vi "UDP dSpace Reveiver.vi"(7 "milliseconds to wait":u32, 8 "error in (no error)":errorcluster, 10 "ENQUE DIRECTLY":refnum<queue>, 11 "UDP Network Connection in":refnum<k16>) -> (0 "error out":errorcluster)   [LabVIEW 2016]
uses:
  Globale Variablen VI/AutonomousMode.vi
  Globale Variablen VI/Global Variables.vi
panel:
  out "value":u32
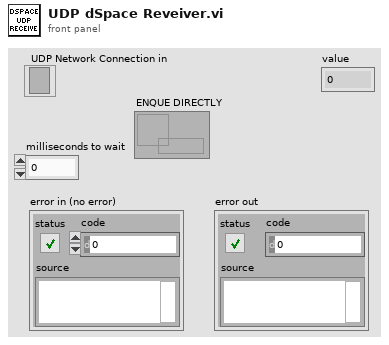
[diagram p1: front panel]
types:
  T1 = enum16{"big-endian, network order", "native, host order", "little-endian"}
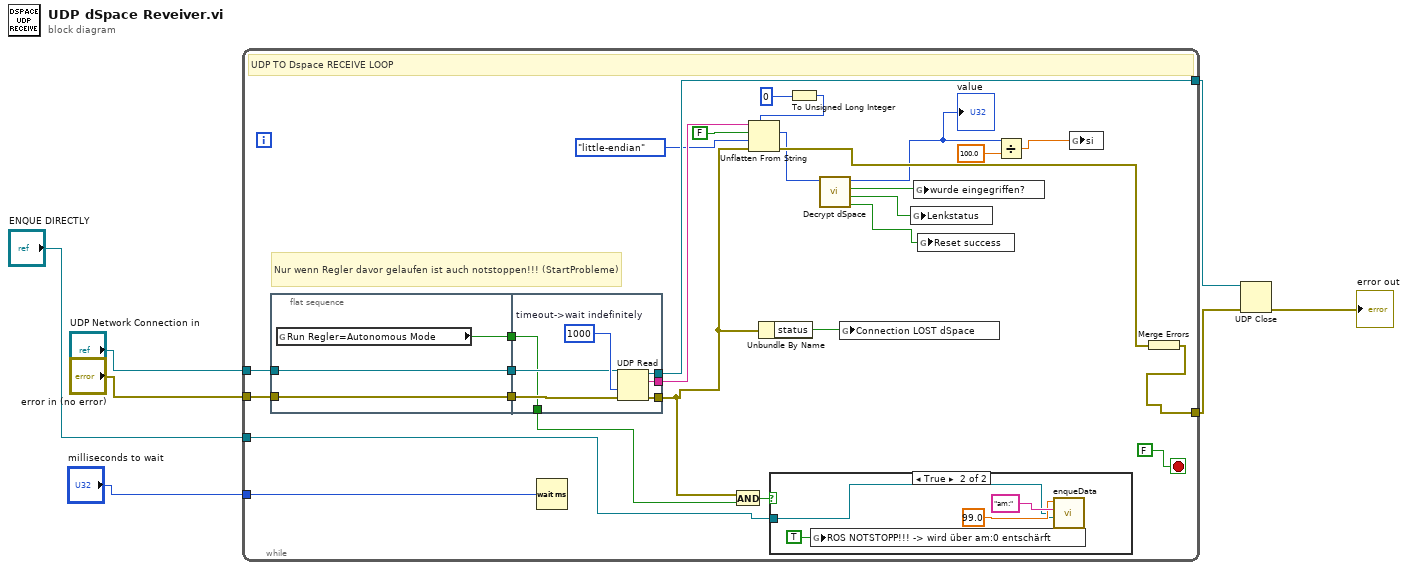
[diagram p0: block diagram]
diagram:
  n1 = while {
    tunnel: [w34] -> w5
    tunnel: [w26] -> w6
    tunnel: "UDP Network Connection in" -> [w33]
    tunnel: "error in (no error)" -> [w32]
    tunnel: "milliseconds to wait" -> [w25]
    tunnel: "ENQUE DIRECTLY" -> [w19]
    stop <- FALSE stop-if-true
    # "Nur wenn Regler davor gelaufen ist auch notstoppen!!! (StartProbleme)"
    # "UDP TO Dspace RECEIVE LOOP"
    n2 = flat-sequence {
      tunnel: w32 -> [w36]
      tunnel: w33 -> [w37]
      tunnel: [w37] -> w11
      tunnel: [w36] -> w10
      tunnel: [w35] -> w8
      tunnel: [w44] -> w34
      tunnel: [w40] -> w31
      tunnel: [w39] -> w14
      tunnel: w11 -> [w42]
      tunnel: w10 -> [w41]
      tunnel: [w38] -> w9
      tunnel: w8 -> [w38]
      frame #0 {
        n3 = global read "AutonomousMode.vi" "Run Regler=Autonomous Mode"() -> (w35:bool)
      }
      frame #1 {
        w43 = 1000  # timeout->wait indefinitely
        n4 = UDP Read(connection ID=w42, timeout ms (25000)=w43, 8:w41) -> (data out=w40:string, error out=w39:errorcluster, 3:w44:refnum<k16>)  [unwired: 3 out]
      }
    }
    n5 = Wait (ms)(milliseconds to wait=w25) -> ()  [unwired: 1 out]
    n6 = And(x=w14, y=w9) -> (x .and. y?=w20:bool)
    n7 = Unbundle By Name(w14) -> ("status"=w13:bool)
    n8 = case shown="True" w20 {
      tunnel: w19 -> [_ w45]
      frame False {
      }
      frame True {
        n9 = global write "AutonomousMode.vi" "ROS NOTSTOPP!!! -> wird über am:0 entschärft"(TRUE ("ROS NOTSTOPP!!! -> wird über am:0 entschärft")) -> ()
        n10 = call "enqueData.vi"("Queue Reference"=w45, "Descriptor"="am:", "Value IN"=99.0) -> ()  [unwired: 8 in, 1 out]
      }
    }
    n11 = To Unsigned Long Integer(number=0) -> (unsigned 32bit integer=w27:u32)
    n12 = Unflatten From String(type=w27, binary string=w31, data includes array or string size? (T)=FALSE, byte order (0:big-endian, network order)=T1."little-endian", error in (no error)=w14) -> (value=w23:u32, error out=w24:errorcluster)  [unwired: 1 out]
    n13 = call "Decrypt dSpace.vi"("Numeric in"=w23) -> ("Reset succesful"=w12:bool, "Lenkstatus"=w21:bool, "wurde eingegriffen?"=w22:bool, "Numeric out"=w16:u32)  [unwired: 7 in]
    "value" <- w16
    n14 = global write "Global Variables.vi" "Connection LOST dSpace"(w13) -> ()
    n15 = global write "Global Variables.vi" "Lenkstatus"(w21) -> ()
    n16 = global write "Global Variables.vi" "wurde eingegriffen?"(w22) -> ()
    n17 = global write "Global Variables.vi" "Reset success"(w12) -> ()
    n18 = Divide(x=w16, y=100.0) -> (x/y=w17:dbl)
    n19 = global write "Global Variables.vi" "si"(w17) -> ()
    n20 = Merge Errors(w24) -> (w26:errorcluster)
  }
  n21 = UDP Close(connection ID=w5, 8:w6) -> (error out=→"error out":errorcluster)  [unwired: 1 out]
